vi "Change-substatus.vi"(9 "Reset errors?":bool, 10 "New status in":T1, 11 "Previous status":T1) -> (2 "New status":T1)   [LabVIEW 2013, in "CameraVision.lvlib" / "CV-Main.lvclass"]
uses:
  CV-Main.lvclass
  UI/Module-states.ctl
  UI/CV-UI.lvclass
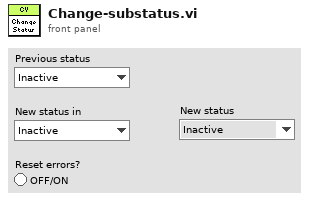
[diagram p1: front panel]
types:
  T1 = typedef "CameraVision.lvlib/CV-UI.lvclass/Module-states.ctl" = enum16{"Inactive", "Active", "Data-loss", "Error", "Simulation", "Synchronizing", "Initialized", "Released"}
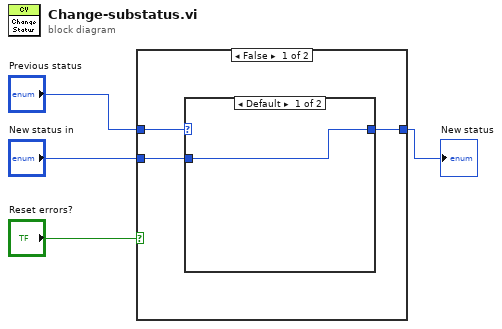
[diagram p0: block diagram]
diagram:
  n1 = case shown="False" "Reset errors?" {
    tunnel: "Previous status" -> [w7 _]
    tunnel: "New status in" -> [w6 w10]
    tunnel: [w5 w10] -> w4
    frame False {
      n2 = case shown="Default" w7 {
        selector: w7 -> [_ w9]
        tunnel: w6 -> [w8 _]
        tunnel: [w8 w9] -> w5
        frame Default {
        }
        frame "Data-loss", "Error" {
        }
      }
    }
    frame True {
    }
  }
  "New status" <- w4
